vi "GUI.vi"() -> ()   [LabVIEW 2016]
panel:
  in  "Oxidizer Error Percent":string
  in  "Fuel Error Percent":string
  in  "Oxidizer Orifice (in)":string
  in  "Oxidizer Pressure (psi)":string
  in  "Fuel Pressure (psi)":string
  in  "Fuel Orifice (in)":string
  in  "Category Selector":T1(tab)
  in  "Fuel":string
  in  "Oxidizer":string
  in  "Desired Eqivalence Ratio":string
  in  "Temperature (K)":string
  in  "Maximum Fuel Pressure (Pa)":string
  in  "Maximum Oxidizer Pressure (Pa)\n 2":string
  in  "Operating Frequency (Hz)":string
  in  "PDE Tube Diameter (m)":string
  in  "PDE Tube Length (m)":string
  in  "Available Orifice Sizes":i32[](listbox)
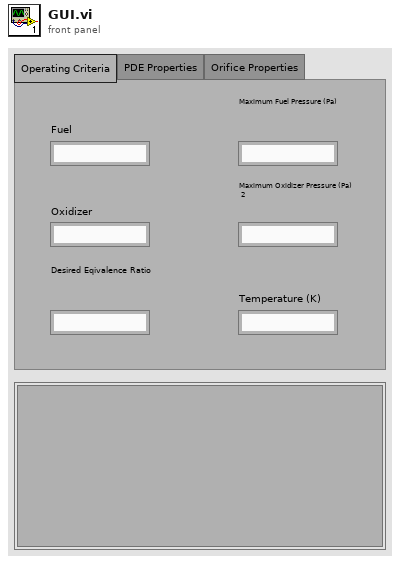
[diagram p1: front panel]
types:
  T1 = enum32{"Operating Criteria", "PDE Properties", "Orifice Properties"}
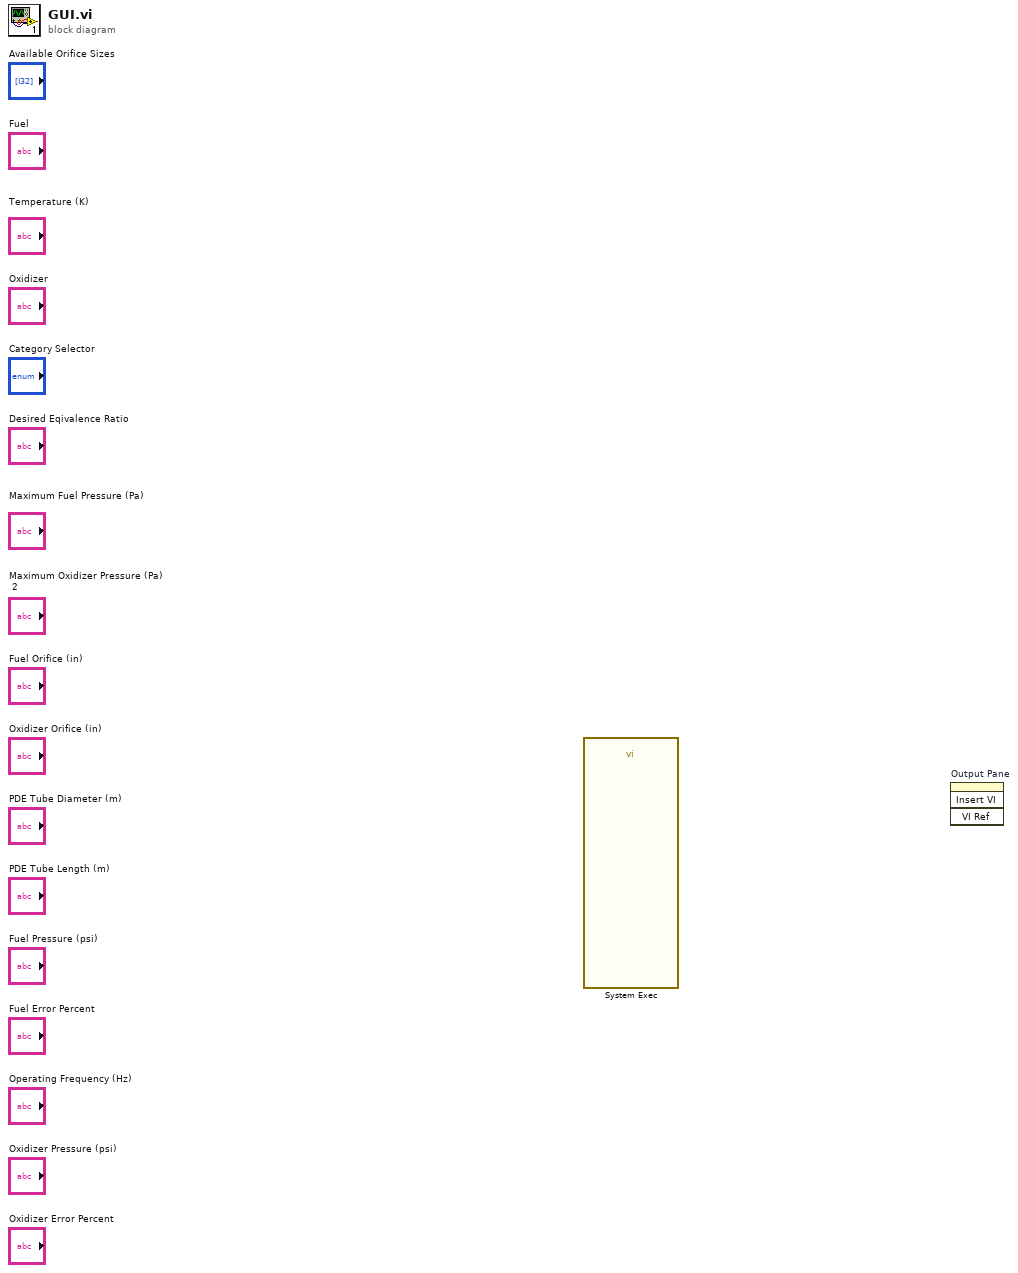
[diagram p0: block diagram]
diagram:
  n1 = call <vilib>:"System Exec.vi"() -> ()  [unwired: 8 in, 4 out]
  n2 = invoke on="Output Pane" class="SubPnl" method="Insert VI"() -> ()  [unwired: 4 in, 4 out]
